vi "RT Driver VI.vi"(6 "Device Clock":string, 9 "Device Inputs FIFO":refnum<k33>, 10 "Device Outputs FIFO":refnum<k33>, 11 "Device Reference":T1 format="%.0x") -> ()   [LabVIEW 2020, in "G5 Regatron Custom Device Engine.lvlib"]
uses:
  G5 Regatron Custom Device Engine.lvlib
  <vilib>/NI VeriStand/Custom Device API/Custom Device Item Ref.ctl
  <vilib>/NI VeriStand/Custom Device API/Custom Device Channel Type.ctl
  <vilib>/Platform/TimedLoop/XDataNode/timing_clust.ctl
  <vilib>/Platform/TimedLoop/XDataNode/nitl_modes.ctl
  <vilib>/Platform/TimedLoop/XDataNode/wakeup.ctl
  Shared/Regatron.G5.Rest Handle.llb/G5.Rest Status.ctl
  Shared/Regatron.G5.Rest System.llb/G5.Rest System Output References Datasource.ctl
  Shared/Regatron.G5.Rest System.llb/G5.Rest System Output Limits.ctl
  Shared/Regatron.G5.Rest System.llb/G5.Rest System Output Limits Datasource.ctl
  Shared/Regatron.G5.Rest System.llb/G5.Rest System Output References.ctl
  Shared/Regatron.G5.Rest System.llb/G5.Rest System Clear Inicidents.ctl
  Shared/Regatron.G5.Rest Config.llb/G5.Rest Sensing Observation References.ctl
  Shared/Regatron.G5.Rest Config.llb/G5.Rest Config Sensing Observation Datasource.ctl
  <userlib>/_OpenG.lib/array/array.llb/Search 1D Array (Boolean)__ogtk.vi
  <vilib>/platform/TimedLoop/XDataNode/XDataNode.xnode
  <vilib>/NI VeriStand/Custom Device API/Custom Device API.lvlib
  <vilib>/NI VeriStand/Custom Device Tools/Custom Device Utility Library/Custom Device Utility Library.lvlib
  <vilib>/Platform/TimedLoop/XDataNode/XDNodeRunTimeDep.lvlib
  Shared/Regatron.G5.Rest.lvlib
panel:
  in  "Initialization Status Notifier":refnum<notifier>
  in  "Status Notifier":refnum<notifier>
  # "Custom Device Template\nv1.0"
  # "Use this template as a starting point for creating a custom device code module. The input controls shown here are specially named controls that the system will use to provide the device loop with data. The controls are not required for the device loop to run. For instance, if the device doesn't produce any output data, then you don't need the Device Outputs FIFO control. If you do use these controls, however, they need to have these exact names to be functional."
  # "The optional status notifier element is used to notify the RT engine of the last state of the custom device, and to indicate the device has completed execution. If this control is not used, a default No Error value is returned to the system when the device finishes execution.\n\nNote: This error state is not checked until the system shuts down. Use an output status channel to send more immediate status values to the system."
  # "This optional input can be used to send the VeriStand Engine the final status of the custom device initalization process. If this control exists on the custom device front panel, the VeriStand Engine will wait for a status update before starting up. If the custom device reports an error, that will abort the execution of the current configuration in the VeriStand Engine.\n\nThis control can be deleted if the custom device does not need to send the initialization status update."
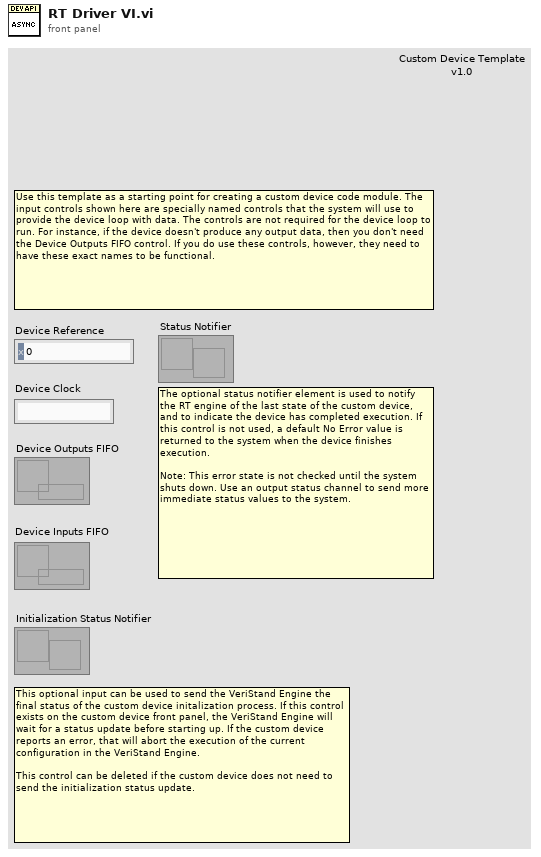
[diagram p1: front panel]
types:
  T1 = typedef "Custom Device API.lvlib/Custom Device Item Ref.ctl" = u64
  T2 = typedef "Custom Device API.lvlib/Custom Device Channel Type.ctl" = enum16{"Input", "Output"}
  T3 = typedef "Custom Device API.lvlib/Custom Device Timed Loop Priority.ctl" = enum32{"Low", "Medium", "High"}
  T4 = typedef "XDNodeRunTimeDep.lvlib/nitl_modes.ctl" = enum32{"No Change", "Process missed periods, maintain original phase", "Discard missed periods, maintain original phase", "Process missed periods, ignore original phase", "Discard missed periods, ignore original phase"}
  T5 = typedef "XDNodeRunTimeDep.lvlib/timing_clust.ctl" = cluster{"Expected End [f-1]":u64, "Actual End [f-1]":u64, "Finished Late? [f-1]":bool, "Expected End [i-1]":u64, "Actual End [i-1]":u64, "Finished Late? [i-1]":bool, "Expected Start [i]":u64, "Actual Start [i]":u64, "Expected Start [f]":u64, "Actual Start [f]":u64, "Source Name":string, "Structure Name":string, "Period":i64, "Deadline":i64, "Offset":i64, "Start":i64, "Priority":i32, "Timeout":i32, "Mode":T4, "Wakeup Reason":T6, "Error":errorcluster, "Source Type":string, "Secondary Source Type":string, "Global End Time":u64, "Global Start Time":u64, "Frame Duration":u64, "Iteration Duration":u64, "Assigned CPU":i32, "I/O Scan Engine Mode":u32}
  T6 = typedef "XDNodeRunTimeDep.lvlib/wakeup.ctl" = enum32{"Normal", "Aborted", "Asynchronous wakeup", "Timing source error", "Timed loop error", "Timeout"}
  T7 = typedef "Regatron.G5.Rest.lvlib/G5.Rest Status.ctl" = enum16{"Read", "Write"}
  T8 = typedef "Regatron.G5.Rest.lvlib/G5.Rest System Output Limits.ctl" = cluster{"Voltage Upper Limit V":sgl, "Voltage Lower Limit V":sgl, "Current Upper Limit A":sgl, "Current Lower Limit A":sgl, "Power Upper Limit W":sgl, "Power Lower Limit W":sgl}
  T9 = typedef "Regatron.G5.Rest.lvlib/G5.Rest System Output References.ctl" = cluster{"Voltage V":sgl, "Current A":sgl, "Power W":sgl, "Load R Ohm":sgl}
  T10 = typedef "Regatron.G5.Rest.lvlib/G5.Rest System Clear Inicidents.ctl" = enum16{"Clear Errors and Warnings", "Clear Warnings", "Clear Errors"}
  T11 = typedef "Regatron.G5.Rest.lvlib/G5.Rest Sensing Observation References.ctl" = cluster{"Voltage Max Level (V)":sgl, "Voltage Max Delay (ms)":sgl}
  T12 = typedef "Regatron.G5.Rest.lvlib/G5.Rest System Output References Datasource.ctl" = enum16{"Voltage", "Current", "Power", "Load Resistance", "ALL"}[]
  T13 = enum16{"Undefined", "PowerUp", "NotReady", "Ready", "VoltageOnPrepare", "VoltageOn", "VoltageOnLeave", "Test", "FirmwareUpdate"}
  T14 = typedef "Regatron.G5.Rest.lvlib/G5.Rest Config Quadrantmode.ctl" = enum16{"Bidirectional", "Q1 Only", "Q4 Only"}
  T15 = typedef "Regatron.G5.Rest.lvlib/G5.Rest System Output Limits Datasource.ctl" = enum16{"Voltage Upper Limit", "Voltage Lower Limit", "Current Upper Limit", "Current Lower Limit", "Power Upper Limit", "Power Lower Limit", "ALL"}[]
  T16 = typedef "Regatron.G5.Rest.lvlib/G5.Rest Config Sensing Observation Datasource.ctl" = enum16{"Voltage Max Level", "Voltage Max Delay", "ALL"}[]
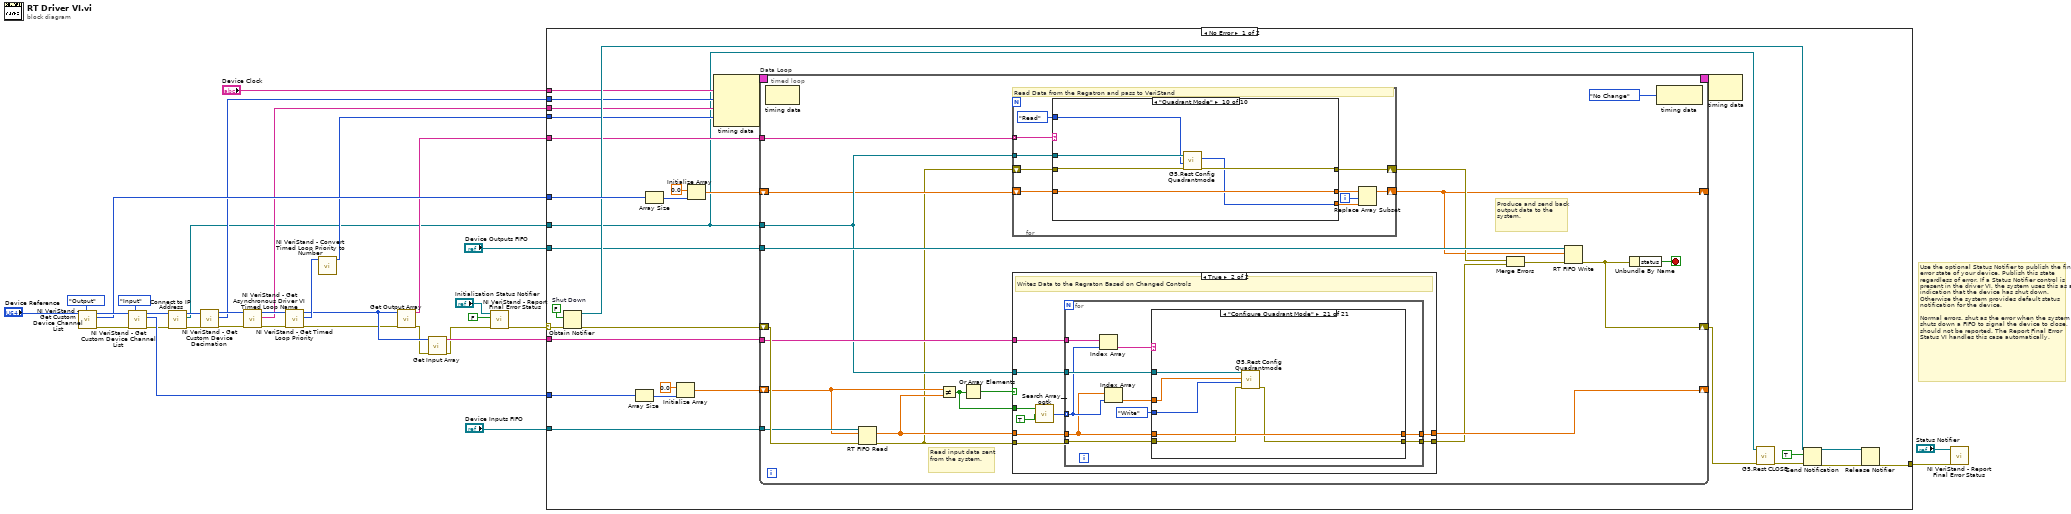
[diagram p0: block diagram]
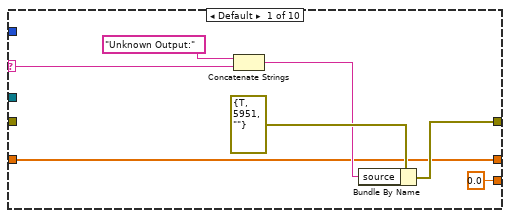
[diagram p2: hidden frame]
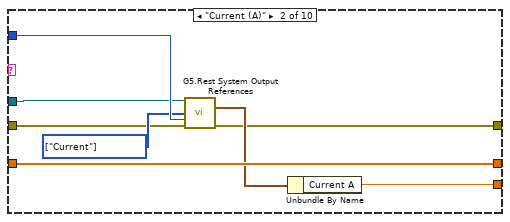
[diagram p3: hidden frame]
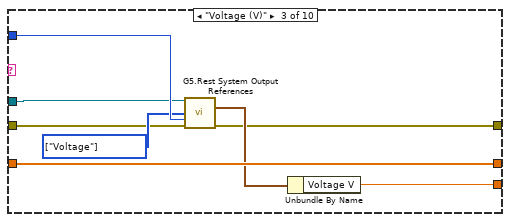
[diagram p4: hidden frame]
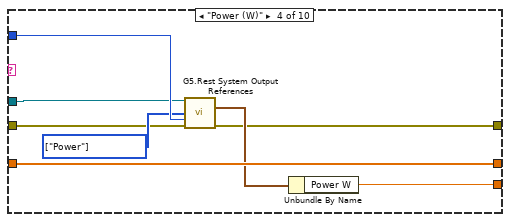
[diagram p5: hidden frame]
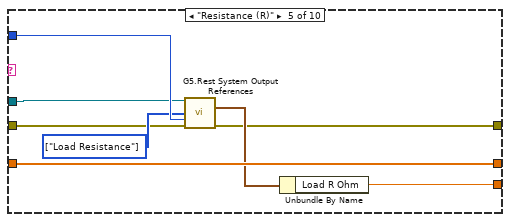
[diagram p6: hidden frame]
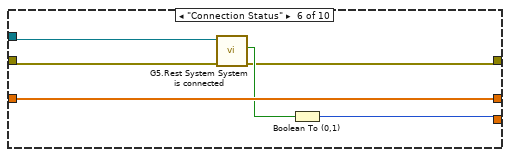
[diagram p7: hidden frame]
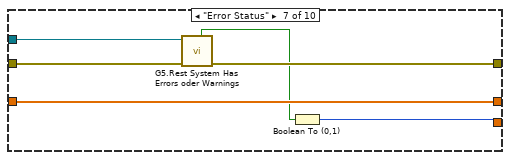
[diagram p8: hidden frame]
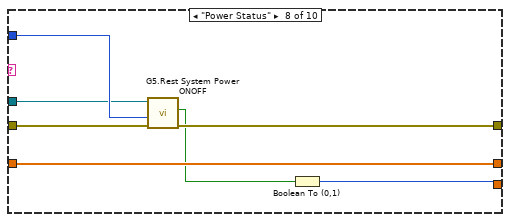
[diagram p9: hidden frame]
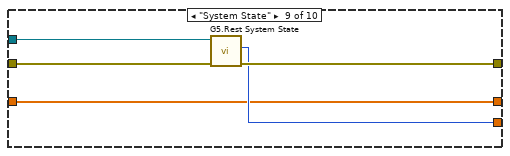
[diagram p10: hidden frame]
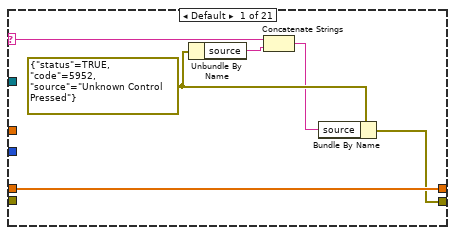
[diagram p12: hidden frame]
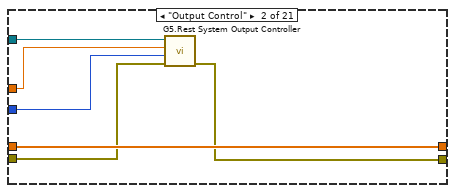
[diagram p13: hidden frame]
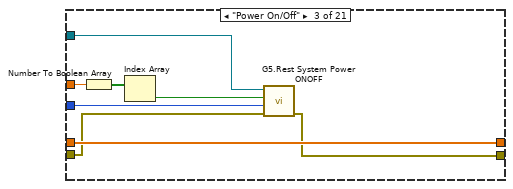
[diagram p14: hidden frame]
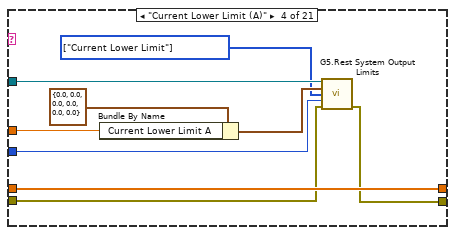
[diagram p15: hidden frame]
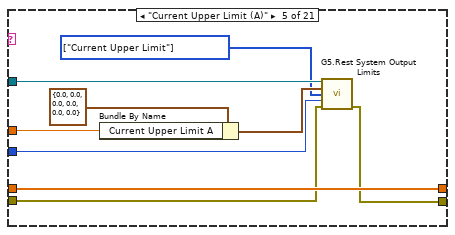
[diagram p16: hidden frame]
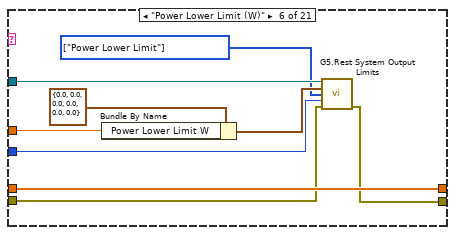
[diagram p17: hidden frame]
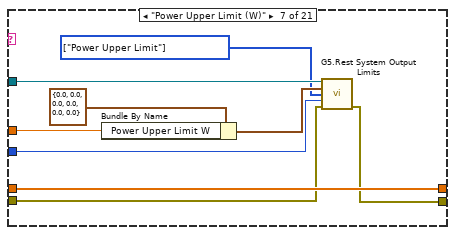
[diagram p18: hidden frame]
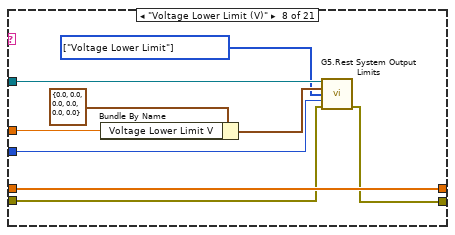
[diagram p19: hidden frame]
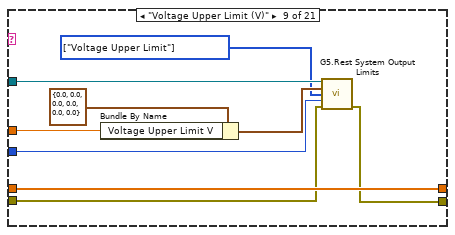
[diagram p20: hidden frame]
diagram:
  # "Use the optional Status Notifier to publish the final error state of your device. Publish this state regardless of error. If a Status Notifier control is present in the driver VI, the system uses this as an indication that the device has shut down. Otherwise the system provides default status notification for the device.\n\nNormal errors, shut as the error when the system shuts down a FIFO to signal the device to close, should not be reported. The Report Final Error Status VI handles this case automatically."
  n1 = call <vilib>:"NI VeriStand - Get Custom Device Channel List.vi"("Channel Type"=Custom_Device_Channel_Type."Output", "Device Ref in"="Device Reference") -> ("error out"=w29:errorcluster, "Specified Channel Ref List"=w26:T1[], "Device Ref out"=w30:T1)  [unwired: 1 in, 6 out]
  n2 = call <vilib>:"NI VeriStand - Get Custom Device Channel List.vi"("Channel Type"=Custom_Device_Channel_Type."Input", "error in (no error)"=w29, "Device Ref in"=w30) -> ("error out"=w20:errorcluster, "Specified Channel Ref List"=w27:T1[], "Device Ref out"=w13:T1)  [unwired: 6 out]
  n3 = call "Connect to IP Address.vi"("error in (no error)"=w20, "Device Ref in"=w13) -> ("error out"=w14:errorcluster, "REST Client out"=w1:refnum<class "REST Client.lvclass">, "Item Ref out"=w12:T1)  [unwired: 7 in]
  n4 = call <vilib>:"NI VeriStand - Get Custom Device Decimation.vi"("error in (no error)"=w14, "Device Ref in"=w12) -> ("error out"=w18:errorcluster, "Decimation"=w10:i32, "Device Ref out"=w19:T1)  [unwired: 7 in]
  n5 = call <vilib>:"NI VeriStand - Get Asynchronous Driver VI Timed Loop Name.vi"("error in (no error)"=w18, "Device Ref in"=w19) -> ("error out"=w17:errorcluster, "Device Timed Loop Name"=w9:string, "Device Ref out"=w16:T1)  [unwired: 7 in]
  n6 = call <vilib>:"NI VeriStand - Get Timed Loop Priority.vi"("error in (no error)"=w17, "Device Ref in"=w16) -> ("error out"=w6:errorcluster, "Priority"=w15:T3, "Device Ref out"=w7:T1)  [unwired: 7 in]
  n7 = call <vilib>:"NI VeriStand - Convert Timed Loop Priority to Number.vi"("Priority"=w15) -> ("Numeric Priority"=w8:i32)  [unwired: 10 in]
  n8 = call "Get Output Array.vi"("error in"=w6, "Device Ref in"=w7) -> ("error out"=w5:errorcluster, "Array"=w4:string[])  [unwired: 8 in]
  n9 = call "Get Input Array.vi"("error in"=w5, "Device Ref in"=w7) -> ("error out"=w2:errorcluster, "Array"=w3:string[])  [unwired: 8 in]
  n10 = call <vilib>:"NI VeriStand - Report Final Error Status.vi"("error in (no error)"=w2, "Filter FIFO & Shutdown Errors (T)"=FALSE ("Filter FIFO Errors (T)"), "Status Notifier"="Initialization Status Notifier") -> ("error out"=w22:errorcluster)  [unwired: 8 out]
  n11 = case shown="No Error" w22 {
    selector: w22 -> [w54 w360]
    tunnel: "Device Outputs FIFO" -> [w46 _]
    tunnel: "Device Inputs FIFO" -> [w48 _]
    tunnel: w27 -> [w60 _]
    tunnel: w26 -> [w59 _]
    tunnel: [w56 w360] -> w24
    tunnel: "Device Clock" -> [w43 _]
    tunnel: w10 -> [w42 _]
    tunnel: w9 -> [w41 _]
    tunnel: w8 -> [w40 _]
    tunnel: w4 -> [w39 _]
    tunnel: w3 -> [w38 _]
    tunnel: w1 -> [w35 _]
    frame No Error {
      w57 = FALSE  # Shut Down
      n12 = Obtain Notifier(notification data type=w57, error in (no error)=w54) -> (notifier out=w55:refnum<notifier>, error out=w45:errorcluster)  [unwired: 2 in, 1 out]
      n13 = Array Size(array=w60) -> (size(s)=w58:i32)
      n14 = Array Size(array=w59) -> (size(s)=w61:i32)
      n15 = Initialize Array(0.0 ("element"), w58) -> (w49:dbl[])
      n16 = Initialize Array(0.0 ("element"), w61) -> (w47:dbl[])
      n17 = node-c288(w43, w42, w41, w40) -> (w51:T5)
      n18 = timed-loop "Data Loop" {
        shift-right: [w82] -> _
        shift-left: w49 -> [w78]
        shift-right: [w79] -> w37
        shift-left: w45 -> [w83]
        shift-right: [w66] -> _
        shift-left: w47 -> [w68]
        tunnel: w46 -> [w81]
        tunnel: w48 -> [w80]
        tunnel: w35 -> [w71]
        tunnel: w38 -> [w77]
        tunnel: w39 -> [w72]
        timing: w51 -> [_]
        timing-out: [_] -> w50
        stop <- w65 stop-if-true
        # "Produce and send back output data to the system."
        # "Read input data sent from the system."
        n19 = node-c288() -> ()  [unwired: 1 in, 1 out]
        n20 = RT FIFO Read(0:w80, 1:w78, 3:w83) -> (9:w74:dbl[], 11:w67:errorcluster)  [unwired: 4 out]
        n21 = Not Equal?(x=w78, y=w74) -> (x != y?=w76:bool[])
        n22 = Or Array Elements(Boolean array=w76) -> (logical OR=w73:bool)
        n23 = for {
          tunnel: w72 -> [w97] mode=indexing
          tunnel: w71 -> [w96]
          shift-right: [w95] -> w69
          shift-left: w67 -> [w93]
          shift-right: [w89] -> w66
          shift-left: w68 -> [w94]
          i -> [w91]
          # "Read Data from the Regatron and pass to VeriStand"
          n24 = case shown="\"Quadrant Mode\"" w97 {
            selector: w97 -> [w99 _ _ _ _ _ _ _ _ _]
            tunnel: w96 -> [_ w106 w114 w122 w130 w140 w146 w152 w160 w166]
            tunnel: w93 -> [_ w107 w115 w123 w131 w139 w145 w151 w159 w164]
            tunnel: [w102 w105 w113 w121 w129 w137 w144 w150 w158 w163] -> w95
            tunnel: w94 -> [w100 w112 w120 w128 w136 w142 w148 w155 w156 w162]
            tunnel: [w100 w112 w120 w128 w136 w142 w148 w155 w156 w162] -> w92
            tunnel: [sgl 0.0 ("Load R Ohm") w110 w118 w126 w134 w141 w147 w154 w157 w161] -> w90
            tunnel: G5.Rest_Status."Read" ("Status") -> [_ w109 w117 w125 w133 _ _ w153 _ w165]
            frame Default {
              n25 = Concatenate Strings("Unknown Output:" ("string"), w99) -> (w103:string)
              n26 = Bundle By Name(cluster=errorcluster {"status"=TRUE, "code"=5951, "source"=""} ("Fehler (Ausgang)"), "source"=w103) -> (w102:errorcluster)
            }
            frame "Current (A)" {
              w108 = T12 [enum."Current"] items=["Voltage", "Current", "Power", "Load Resistance", "ALL"] ("Datasource")
              n27 = call "G5.Rest System Output References .vi"("G5 WEB API (Eingang)"=w106, "Datasource"=w108, "Status"=w109, "Fehler (Eingang, kein Fehler)"=w107) -> ("GET Output Reference"=w111:T9, "Fehler (Ausgang)"=w105:errorcluster)  [unwired: 9 in, 1 out]
              n28 = Unbundle By Name(w111) -> ("Current A"=w110:sgl)
            }
            frame "Voltage (V)" {
              w116 = T12 [enum."Voltage"] items=["Voltage", "Current", "Power", "Load Resistance", "ALL"] ("Datasource")
              n29 = call "G5.Rest System Output References .vi"("G5 WEB API (Eingang)"=w114, "Datasource"=w116, "Status"=w117, "Fehler (Eingang, kein Fehler)"=w115) -> ("GET Output Reference"=w119:T9, "Fehler (Ausgang)"=w113:errorcluster)  [unwired: 9 in, 1 out]
              n30 = Unbundle By Name(w119) -> ("Voltage V"=w118:sgl)
            }
            frame "Power (W)" {
              w124 = T12 [enum."Power"] items=["Voltage", "Current", "Power", "Load Resistance", "ALL"] ("Datasource")
              n31 = call "G5.Rest System Output References .vi"("G5 WEB API (Eingang)"=w122, "Datasource"=w124, "Status"=w125, "Fehler (Eingang, kein Fehler)"=w123) -> ("GET Output Reference"=w127:T9, "Fehler (Ausgang)"=w121:errorcluster)  [unwired: 9 in, 1 out]
              n32 = Unbundle By Name(w127) -> ("Power W"=w126:sgl)
            }
            frame "Resistance (R)" {
              w132 = T12 [enum."Load Resistance"] items=["Voltage", "Current", "Power", "Load Resistance", "ALL"] ("Datasource")
              n33 = call "G5.Rest System Output References .vi"("G5 WEB API (Eingang)"=w130, "Datasource"=w132, "Status"=w133, "Fehler (Eingang, kein Fehler)"=w131) -> ("GET Output Reference"=w135:T9, "Fehler (Ausgang)"=w129:errorcluster)  [unwired: 9 in, 1 out]
              n34 = Unbundle By Name(w135) -> ("Load R Ohm"=w134:sgl)
            }
            frame "Connection Status" {
              n35 = call "G5.Rest System System is connected.vi"("Fehler (Eingang, kein Fehler)"=w139, "G5 WEB API (Eingang)"=w140) -> ("Fehler (Ausgang)"=w137:errorcluster, "System is connected"=w138:bool)  [unwired: 7 in, 1 out]
              n36 = Boolean To (0,1)(Boolean=w138) -> (0, 1=w141:i16)
            }
            frame "Error Status" {
              n37 = call "G5.Rest System Has Errors oder Warnings.vi"("Fehler (Eingang, kein Fehler)"=w145, "G5 WEB API (Eingang)"=w146) -> ("Fehler (Ausgang)"=w144:errorcluster, "System has Errors or Warnings"=w143:bool)  [unwired: 5 in, 3 out]
              n38 = Boolean To (0,1)(Boolean=w143) -> (0, 1=w147:i16)
            }
            frame "Power Status" {
              n39 = call "G5.Rest System Power ONOFF.vi"("Fehler (Eingang, kein Fehler)"=w151, "Status"=w153, "G5 WEB API (Eingang)"=w152) -> ("Fehler (Ausgang)"=w150:errorcluster, "Get Power OFF/ON"=w149:bool)  [unwired: 6 in, 1 out]
              n40 = Boolean To (0,1)(Boolean=w149) -> (0, 1=w154:i16)
            }
            frame "System State" {
              n41 = call "G5.Rest System State.vi"("Fehler (Eingang, kein Fehler)"=w159, "G5 WEB API (Eingang)"=w160) -> ("Fehler (Ausgang)"=w158:errorcluster, "GET State"=w157:T13)  [unwired: 7 in, 1 out]
            }
            frame "Quadrant Mode" {
              n42 = call "G5.Rest Config Quadrantmode.vi"("Fehler (Eingang, kein Fehler)"=w164, "Status"=w165, "G5 WEB API (Eingang)"=w166) -> ("Fehler (Ausgang)"=w163:errorcluster, "GET Quadrant Mode"=w161:T14)  [unwired: 6 in, 1 out]
            }
          }
          n43 = Replace Array Subset(array=w92, new element=w90, index=w91) -> (w89:dbl[])
        }
        n44 = case shown="True" w73 {
          tunnel: w71 -> [_ w177]
          tunnel: w67 -> [w168 w176]
          tunnel: w76 -> [_ w175]
          tunnel: w77 -> [_ w172]
          tunnel: [w168 w171] -> w75
          tunnel: w74 -> [w167 w170]
          tunnel: [w167 w169] -> w82
          frame False {
          }
          frame True {
            # "Writes Data to the Regraton Based on Changed Controls"
            n45 = call-poly <userlib>:"Search Array__ogtk.vi"("Array"=w175, "Element Data"=TRUE) -> ("Indices of Elements"=w173:i32[])  [unwired: 7 in]
            n46 = for {
              tunnel: w177 -> [w187]
              tunnel: w176 -> [w186]
              tunnel: w173 -> [w183] mode=indexing
              tunnel: w172 -> [w185]
              tunnel: [w181] -> w171
              tunnel: w170 -> [w180]
              tunnel: [w179] -> w169
              n47 = Index Array(array=w185, index=w183) -> (element=w184:string)
              n48 = Index Array(array=w180, index=w183) -> (element=w182:dbl)
              n49 = case shown="\"Configure Quadrant Mode\"" w184 {
                selector: w184 -> [w189 _ _ _ _ _ _ _ _ _ _ _ _ _ _ _ _ _ _ _ _]
                tunnel: w187 -> [_ w198 w202 w215 w224 w233 w242 w251 w260 w269 w278 w287 w296 w301 w309 w315 w323 w327 w336 w345 w351]
                tunnel: w186 -> [_ w197 w203 w210 w219 w228 w237 w246 w255 w268 w277 w286 w295 w300 w308 w312 w322 w326 w335 w344 w350]
                tunnel: w182 -> [_ w195 w205 w212 w221 w230 w239 w248 w257 w263 w272 w281 w290 _ w305 w314 w318 w330 w339 _ w348]
                tunnel: [w191 w194 w201 w209 w218 w227 w236 w245 w254 w265 w274 w283 w292 w299 w303 w311 w317 w325 w334 w343 w347] -> w181
                tunnel: w180 -> [w193 w199 w207 w216 w225 w234 w243 w252 w261 w270 w279 w288 w297 w302 w310 w316 w324 w333 w342 w346 w352]
                tunnel: [w193 w199 w207 w216 w225 w234 w243 w252 w261 w270 w279 w288 w297 w302 w310 w316 w324 w333 w342 w346 w352] -> w179
                tunnel: G5.Rest_Status."Write" ("Status") -> [_ w196 w200 w214 w223 w232 w241 w250 w259 w267 w276 w285 w294 _ w307 w313 w321 w329 w338 _ w349]
                frame Default {
                  w192 = errorcluster {"status"=TRUE, "code"=5952, "source"="Unknown Control Pressed"} ("Fehler (Ausgang)")
                  n50 = Unbundle By Name(w192) -> ("source"=w190:string)
                  n51 = Concatenate Strings(w189, w190) -> (w188:string)
                  n52 = Bundle By Name(cluster=w192, "source"=w188) -> (w191:errorcluster)
                }
                frame "Output Control" {
                  n53 = call "G5.Rest System Output Controller.vi"("Fehler (Eingang, kein Fehler)"=w197, "Status"=w196, "SET Output Control"=w195, "G5 WEB API (Eingang)"=w198) -> ("Fehler (Ausgang)"=w194:errorcluster)  [unwired: 5 in, 2 out]
                }
                frame "Power On/Off" {
                  n54 = Number To Boolean Array(number=w205) -> (Boolean array=w206:bool[])
                  n55 = Index Array(array=w206) -> (element=w204:bool)  [unwired: 1 in]
                  n56 = call "G5.Rest System Power ONOFF.vi"("Fehler (Eingang, kein Fehler)"=w203, "Status"=w200, "Power OFF/ON"=w204, "G5 WEB API (Eingang)"=w202) -> ("Fehler (Ausgang)"=w201:errorcluster)  [unwired: 5 in, 2 out]
                }
                frame "Current Lower Limit (A)" {
                  w208 = T15 [enum."Current Lower Limit"] items=["Voltage Upper Limit", "Voltage Lower Limit", "Current Upper Limit", "Current Lower Limit", "Power Upper Limit", "Power Lower Limit", "ALL"] ("Datasource")
                  n57 = Bundle By Name(cluster=T8 {"Voltage Upper Limit V"=0.0, "Voltage Lower Limit V"=0.0, "Current Upper Limit A"=0.0, "Current Lower Limit A"=0.0, "Power Upper Limit W"=0.0, "Power Lower Limit W"=0.0} ("SET Output Limit"), "Current Lower Limit A"=w212) -> (w211:T8)
                  n58 = call "G5.Rest System Output Limits.vi"("G5 WEB API (Eingang)"=w215, "SET Output Limit"=w211, "Datasource"=w208, "Status"=w214, "Fehler (Eingang, kein Fehler)"=w210) -> ("Fehler (Ausgang)"=w209:errorcluster)  [unwired: 8 in, 2 out]
                }
                frame "Current Upper Limit (A)" {
                  w217 = T15 [enum."Current Upper Limit"] items=["Voltage Upper Limit", "Voltage Lower Limit", "Current Upper Limit", "Current Lower Limit", "Power Upper Limit", "Power Lower Limit", "ALL"] ("Datasource")
                  n59 = Bundle By Name(cluster=T8 {"Voltage Upper Limit V"=0.0, "Voltage Lower Limit V"=0.0, "Current Upper Limit A"=0.0, "Current Lower Limit A"=0.0, "Power Upper Limit W"=0.0, "Power Lower Limit W"=0.0} ("SET Output Limit"), "Current Upper Limit A"=w221) -> (w220:T8)
                  n60 = call "G5.Rest System Output Limits.vi"("G5 WEB API (Eingang)"=w224, "SET Output Limit"=w220, "Datasource"=w217, "Status"=w223, "Fehler (Eingang, kein Fehler)"=w219) -> ("Fehler (Ausgang)"=w218:errorcluster)  [unwired: 8 in, 2 out]
                }
                frame "Power Lower Limit (W)" {
                  w226 = T15 [enum."Power Lower Limit"] items=["Voltage Upper Limit", "Voltage Lower Limit", "Current Upper Limit", "Current Lower Limit", "Power Upper Limit", "Power Lower Limit", "ALL"] ("Datasource")
                  n61 = Bundle By Name(cluster=T8 {"Voltage Upper Limit V"=0.0, "Voltage Lower Limit V"=0.0, "Current Upper Limit A"=0.0, "Current Lower Limit A"=0.0, "Power Upper Limit W"=0.0, "Power Lower Limit W"=0.0} ("SET Output Limit"), "Power Lower Limit W"=w230) -> (w229:T8)
                  n62 = call "G5.Rest System Output Limits.vi"("G5 WEB API (Eingang)"=w233, "SET Output Limit"=w229, "Datasource"=w226, "Status"=w232, "Fehler (Eingang, kein Fehler)"=w228) -> ("Fehler (Ausgang)"=w227:errorcluster)  [unwired: 8 in, 2 out]
                }
                frame "Power Upper Limit (W)" {
                  w235 = T15 [enum."Power Upper Limit"] items=["Voltage Upper Limit", "Voltage Lower Limit", "Current Upper Limit", "Current Lower Limit", "Power Upper Limit", "Power Lower Limit", "ALL"] ("Datasource")
                  n63 = Bundle By Name(cluster=T8 {"Voltage Upper Limit V"=0.0, "Voltage Lower Limit V"=0.0, "Current Upper Limit A"=0.0, "Current Lower Limit A"=0.0, "Power Upper Limit W"=0.0, "Power Lower Limit W"=0.0} ("SET Output Limit"), "Power Upper Limit W"=w239) -> (w238:T8)
                  n64 = call "G5.Rest System Output Limits.vi"("G5 WEB API (Eingang)"=w242, "SET Output Limit"=w238, "Datasource"=w235, "Status"=w241, "Fehler (Eingang, kein Fehler)"=w237) -> ("Fehler (Ausgang)"=w236:errorcluster)  [unwired: 8 in, 2 out]
                }
                frame "Voltage Lower Limit (V)" {
                  w244 = T15 [enum."Voltage Lower Limit"] items=["Voltage Upper Limit", "Voltage Lower Limit", "Current Upper Limit", "Current Lower Limit", "Power Upper Limit", "Power Lower Limit", "ALL"] ("Datasource")
                  n65 = Bundle By Name(cluster=T8 {"Voltage Upper Limit V"=0.0, "Voltage Lower Limit V"=0.0, "Current Upper Limit A"=0.0, "Current Lower Limit A"=0.0, "Power Upper Limit W"=0.0, "Power Lower Limit W"=0.0} ("SET Output Limit"), "Voltage Lower Limit V"=w248) -> (w247:T8)
                  n66 = call "G5.Rest System Output Limits.vi"("G5 WEB API (Eingang)"=w251, "SET Output Limit"=w247, "Datasource"=w244, "Status"=w250, "Fehler (Eingang, kein Fehler)"=w246) -> ("Fehler (Ausgang)"=w245:errorcluster)  [unwired: 8 in, 2 out]
                }
                frame "Voltage Upper Limit (V)" {
                  w253 = T15 [enum."Voltage Upper Limit"] items=["Voltage Upper Limit", "Voltage Lower Limit", "Current Upper Limit", "Current Lower Limit", "Power Upper Limit", "Power Lower Limit", "ALL"] ("Datasource")
                  n67 = Bundle By Name(cluster=T8 {"Voltage Upper Limit V"=0.0, "Voltage Lower Limit V"=0.0, "Current Upper Limit A"=0.0, "Current Lower Limit A"=0.0, "Power Upper Limit W"=0.0, "Power Lower Limit W"=0.0} ("SET Output Limit"), "Voltage Upper Limit V"=w257) -> (w256:T8)
                  n68 = call "G5.Rest System Output Limits.vi"("G5 WEB API (Eingang)"=w260, "SET Output Limit"=w256, "Datasource"=w253, "Status"=w259, "Fehler (Eingang, kein Fehler)"=w255) -> ("Fehler (Ausgang)"=w254:errorcluster)  [unwired: 8 in, 2 out]
                }
                frame "Current (A)" {
                  w266 = T12 [enum."Current"] items=["Voltage", "Current", "Power", "Load Resistance", "ALL"] ("Datasource")
                  n69 = Bundle By Name(cluster=T9 {"Voltage V"=0.0, "Current A"=0.0, "Power W"=0.0, "Load R Ohm"=0.0} ("SET Output Reference"), "Current A"=w263) -> (w262:T9)
                  n70 = call "G5.Rest System Output References .vi"("G5 WEB API (Eingang)"=w269, "SET Output Reference"=w262, "Datasource"=w266, "Status"=w267, "Fehler (Eingang, kein Fehler)"=w268) -> ("Fehler (Ausgang)"=w265:errorcluster)  [unwired: 8 in, 2 out]
                }
                frame "Power (W)" {
                  w275 = T12 [enum."Power"] items=["Voltage", "Current", "Power", "Load Resistance", "ALL"] ("Datasource")
                  n71 = Bundle By Name(cluster=T9 {"Voltage V"=0.0, "Current A"=0.0, "Power W"=0.0, "Load R Ohm"=0.0} ("SET Output Reference"), "Power W"=w272) -> (w271:T9)
                  n72 = call "G5.Rest System Output References .vi"("G5 WEB API (Eingang)"=w278, "SET Output Reference"=w271, "Datasource"=w275, "Status"=w276, "Fehler (Eingang, kein Fehler)"=w277) -> ("Fehler (Ausgang)"=w274:errorcluster)  [unwired: 8 in, 2 out]
                }
                frame "Resistance (R)" {
                  w284 = T12 [enum."Load Resistance"] items=["Voltage", "Current", "Power", "Load Resistance", "ALL"] ("Datasource")
                  n73 = Bundle By Name(cluster=T9 {"Voltage V"=0.0, "Current A"=0.0, "Power W"=0.0, "Load R Ohm"=0.0} ("SET Output Reference"), "Load R Ohm"=w281) -> (w280:T9)
                  n74 = call "G5.Rest System Output References .vi"("G5 WEB API (Eingang)"=w287, "SET Output Reference"=w280, "Datasource"=w284, "Status"=w285, "Fehler (Eingang, kein Fehler)"=w286) -> ("Fehler (Ausgang)"=w283:errorcluster)  [unwired: 8 in, 2 out]
                }
                frame "Voltage (V)" {
                  w293 = T12 [enum."Voltage"] items=["Voltage", "Current", "Power", "Load Resistance", "ALL"] ("Datasource")
                  n75 = Bundle By Name(cluster=T9 {"Voltage V"=0.0, "Current A"=0.0, "Power W"=0.0, "Load R Ohm"=0.0} ("SET Output Reference"), "Voltage V"=w290) -> (w289:T9)
                  n76 = call "G5.Rest System Output References .vi"("G5 WEB API (Eingang)"=w296, "SET Output Reference"=w289, "Datasource"=w293, "Status"=w294, "Fehler (Eingang, kein Fehler)"=w295) -> ("Fehler (Ausgang)"=w292:errorcluster)  [unwired: 8 in, 2 out]
                }
                frame "Clear Error" {
                  n77 = call "G5.Rest System Clear Inicidents.vi"("Fehler (Eingang, kein Fehler)"=w300, "Clear Inicidents"=G5.Rest_System_Clear_Inicidents."Clear Errors and Warnings", "G5 WEB API (Eingang)"=w301) -> ("Fehler (Ausgang)"=w299:errorcluster)  [unwired: 7 in, 1 out]
                }
                frame "Sense Enable" {
                  n78 = Number To Boolean Array(number=w305) -> (Boolean array=w306:bool[])
                  n79 = Index Array(array=w306) -> (element=w304:bool)  [unwired: 1 in]
                  n80 = call "G5.Rest Config Sensing Enable.vi"("Fehler (Eingang, kein Fehler)"=w308, "Status"=w307, "SET Voltage Sensing Enable"=w304, "G5 WEB API (Eingang)"=w309) -> ("Fehler (Ausgang)"=w303:errorcluster)  [unwired: 5 in, 2 out]
                }
                frame "Sense Max Voltage Compensation (V)" {
                  n81 = call "G5.Rest Config Sensing Compensation.vi"("Fehler (Eingang, kein Fehler)"=w312, "Status"=w313, "SET Sense Max Voltage Compensation"=w314, "G5 WEB API (Eingang)"=w315) -> ("Fehler (Ausgang)"=w311:errorcluster)  [unwired: 5 in, 2 out]
                }
                frame "Sense Observation Enable" {
                  n82 = Number To Boolean Array(number=w318) -> (Boolean array=w319:bool[])
                  n83 = Index Array(array=w319) -> (element=w320:bool)  [unwired: 1 in]
                  n84 = call "G5.Rest Config Sensing Observing Enable.vi"("Fehler (Eingang, kein Fehler)"=w322, "Status"=w321, "SET Sensing Observation Enable"=w320, "G5 WEB API (Eingang)"=w323) -> ("Fehler (Ausgang)"=w317:errorcluster)  [unwired: 5 in, 2 out]
                }
                frame "Sense Observation Voltage Max Level (V)" {
                  w328 = T16 [enum."Voltage Max Level"] items=["Voltage Max Level", "Voltage Max Delay", "ALL"] ("Datasource")
                  n85 = Bundle By Name(cluster=T11 {"Voltage Max Level (V)"=0.0, "Voltage Max Delay (ms)"=0.0} ("SET Sensing Observation References"), "Voltage Max Level (V)"=w330) -> (w331:T11)
                  n86 = call "G5.Rest Config Sensing Observation References.vi"("G5 WEB API (Eingang)"=w327, "SET Sensing Observation References"=w331, "Datasource"=w328, "Status"=w329, "Fehler (Eingang, kein Fehler)"=w326) -> ("Fehler (Ausgang)"=w325:errorcluster)  [unwired: 8 in, 2 out]
                }
                frame "Sense Observation Voltage Max Delay (ms)" {
                  w337 = T16 [enum."Voltage Max Delay"] items=["Voltage Max Level", "Voltage Max Delay", "ALL"] ("Datasource")
                  n87 = Bundle By Name(cluster=T11 {"Voltage Max Level (V)"=0.0, "Voltage Max Delay (ms)"=0.0} ("SET Sensing Observation References"), "Voltage Max Delay (ms)"=w339) -> (w340:T11)
                  n88 = call "G5.Rest Config Sensing Observation References.vi"("G5 WEB API (Eingang)"=w336, "SET Sensing Observation References"=w340, "Datasource"=w337, "Status"=w338, "Fehler (Eingang, kein Fehler)"=w335) -> ("Fehler (Ausgang)"=w334:errorcluster)  [unwired: 8 in, 2 out]
                }
                frame "Hardware Reset" {
                  n89 = call "G5.Rest System Hardware Reset.vi"("Fehler (Eingang, kein Fehler)"=w344, "G5 WEB API (Eingang)"=w345) -> ("Fehler (Ausgang)"=w343:errorcluster)  [unwired: 8 in, 1 out]
                }
                frame "Configure Quadrant Mode" {
                  n90 = call "G5.Rest Config Quadrantmode.vi"("Fehler (Eingang, kein Fehler)"=w350, "Status"=w349, "SET Quadrant Mode"=w348, "G5 WEB API (Eingang)"=w351) -> ("Fehler (Ausgang)"=w347:errorcluster)  [unwired: 5 in, 2 out]
                }
              }
            }
          }
        }
        n91 = Merge Errors(w69, w75) -> (w70:errorcluster)
        n92 = RT FIFO Write(0:w81, 1:w66, 3:w70) -> (11:w79:errorcluster)  [unwired: 1 in, 4 out]
        n93 = Unbundle By Name(w79) -> ("status"=w65:bool)
        n94 = node-c288(nitl_modes."No Change" ("Mode")) -> ()  [unwired: 1 out]
      }
      n95 = node-c288(w50) -> ()  [unwired: 1 out]
      n96 = call "G5.Rest CLOSE.vi"("Fehler (Eingang, kein Fehler)"=w37, "G5 WEB API"=w35) -> ("error out"=w36:errorcluster)  [unwired: 9 in]
      n97 = Send Notification(notification=TRUE, notifier=w55, error in (no error)=w36) -> (notifier out=w53:refnum<notifier>, error out=w44:errorcluster)
      n98 = Release Notifier(notifier=w53, error in (no error)=w44) -> (error out=w56:errorcluster)  [unwired: 1 in, 2 out]
    }
    frame Error {
    }
  }
  n99 = call <vilib>:"NI VeriStand - Report Final Error Status.vi"("error in (no error)"=w24, "Status Notifier"="Status Notifier") -> ()  [unwired: 1 in, 9 out]
